vi "Set Exp to test.vi"(0 "Test Information":T1={"Exp Name"="Cold Switching", "Lot"="0233A", "Wafer"="15", "Die Type"="L22", "Die X "="6", "Die Y"="8", "Exp"="1", "Die X_Y"="8"}, 5 "Experiments":T3={"Exp 1"={"P2_Sweep_Stop_V"=36.0, "P2_Sweep_Step_V"=1.0, "Experiment Name"="", "Resistance Threshold"=1.0, "P1_Fixed_Voltage"=36.0, "P2_Sweep_Start_V"=36.0}, "Exp 3"={"P2_Sweep_Stop_V"=36.0, "P2_Sweep_Step_V"=1.0, "Experiment Name"="", "Resistance Threshold"=1.0, "P1_Fixed_Voltage"=36.0, "P2_Sweep_Start_V"=36.0}, "Exp 2"={"P2_Sweep_Stop_V"=36.0, "P2_Sweep_Step_V"=1.0, "Experiment Name"="", "Resistance Threshold"=1.0, "P1_Fixed_Voltage"=36.0, "P2_Sweep_Start_V"=36.0}, "Exp 4"={"P2_Sweep_Stop_V"=36.0, "P2_Sweep_Step_V"=1.0, "Experiment Name"="", "Resistance Threshold"=1.0, "P1_Fixed_Voltage"=36.0, "P2_Sweep_Start_V"=36.0}}, 11 "Error In":errorcluster) -> (4 "Selected Exp Settings":T2={"P2_Sweep_Stop_V"=36.0, "P2_Sweep_Step_V"=1.0, "Experiment Name"="", "Resistance Threshold"=1.0, "P1_Fixed_Voltage"=36.0, "P2_Sweep_Start_V"=36.0}, 6 "Test Information Out":T1={"Exp Name"="Cold Switching", "Lot"="0233A", "Wafer"="15", "Die Type"="L22", "Die X "="6", "Die Y"="8", "Exp"="1", "Die X_Y"="8"}, 15 "Error Out":errorcluster)   [LabVIEW 2013]
uses:
  Controls/Multiple Exp Setup.ctl
  Controls/Individual User Inputs.ctl
  Controls/Test Information.ctl
panel:
  # "Test Settings"
  # "Make the Stop and Step Negative \nfor negative sweep"
  # "Calculation Settings"
  # "Test Settings"
  # "Make the Stop and Step Negative \nfor negative sweep"
  # "Calculation Settings"
  # "Test Settings"
  # "Make the Stop and Step Negative \nfor negative sweep"
  # "Calculation Settings"
  # "Test Settings"
  # "Make the Stop and Step Negative \nfor negative sweep"
  # "Calculation Settings"
  # "Test Settings"
  # "Make the Stop and Step Negative \nfor negative sweep"
  # "Calculation Settings"
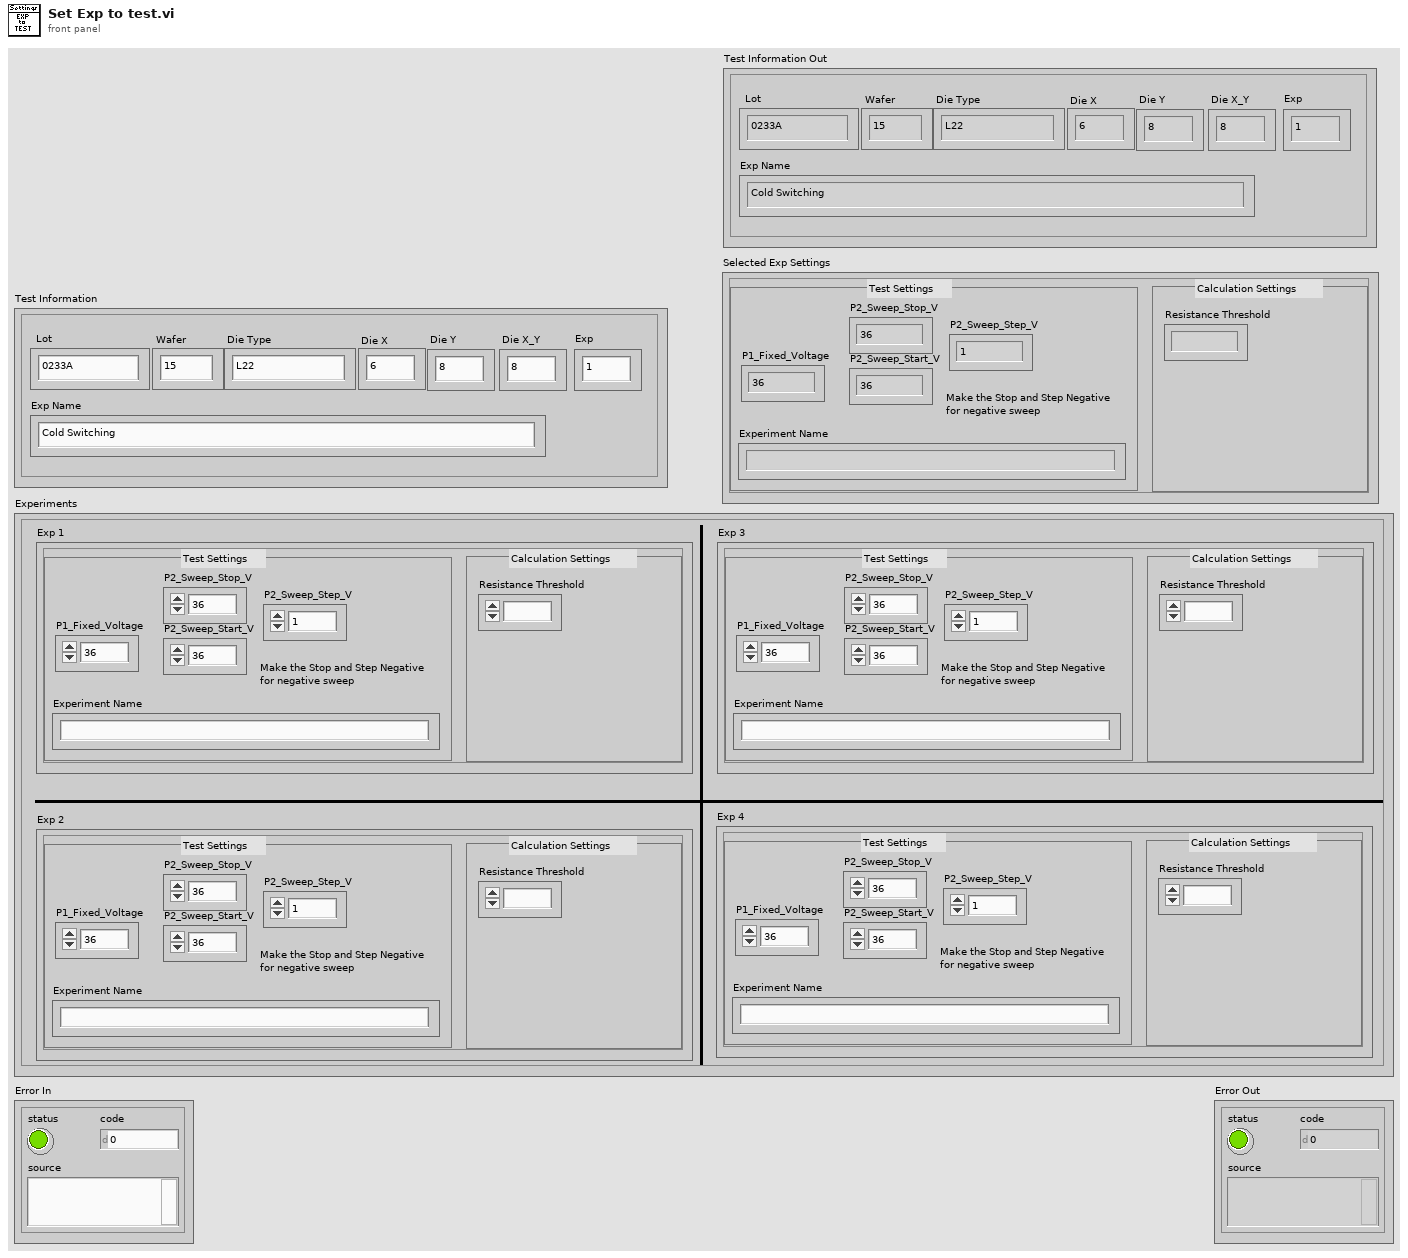
[diagram p1: front panel]
types:
  T1 = typedef "Test Information.ctl" = cluster{"Exp Name":string, "Lot":string, "Wafer":string, "Die Type":string, "Die X ":string, "Die Y":string, "Exp":string, "Die X_Y":string}
  T2 = typedef "Individual User Inputs.ctl" = cluster{"P2_Sweep_Stop_V":dbl, "P2_Sweep_Step_V":dbl, "Experiment Name":string, "Resistance Threshold":dbl, "P1_Fixed_Voltage":dbl, "P2_Sweep_Start_V":dbl}
  T3 = typedef "Multiple Exp Setup.ctl" = cluster{"Exp 1":T2, "Exp 3":T2, "Exp 2":T2, "Exp 4":T2}
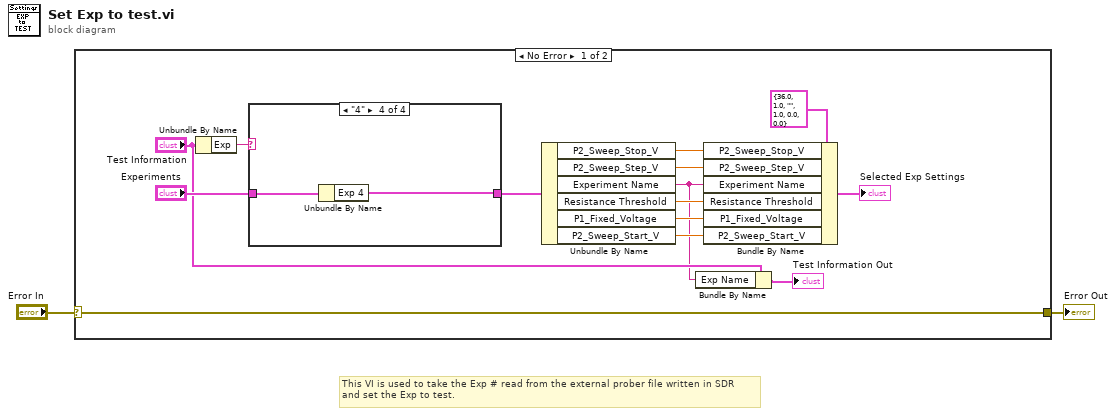
[diagram p0: block diagram]
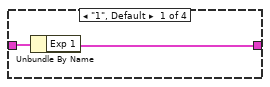
[diagram p2: hidden frame]
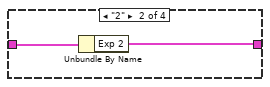
[diagram p3: hidden frame]
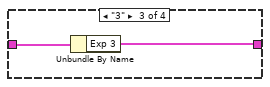
[diagram p4: hidden frame]
diagram:
  # "This VI is used to take the Exp # read from the external prober file written in SDR\nand set the Exp to test."
  n1 = case shown="No Error" "Error In" {
    selector: "Error In" -> [w12 w25]
    tunnel: [w12 w25] -> w1
    frame No Error {
      n2 = Unbundle By Name("Test Information") -> ("Exp"=w16:string)
      n3 = case shown="\"4\"" w16 {
        tunnel: "Experiments" -> [w18 w20 w22 w24]
        tunnel: [w17 w19 w21 w23] -> w4
        frame "1", Default {
          n4 = Unbundle By Name(w18) -> ("Exp 1"=w17:T2)
        }
        frame "2" {
          n5 = Unbundle By Name(w20) -> ("Exp 2"=w19:T2)
        }
        frame "3" {
          n6 = Unbundle By Name(w22) -> ("Exp 3"=w21:T2)
        }
        frame "4" {
          n7 = Unbundle By Name(w24) -> ("Exp 4"=w23:T2)
        }
      }
      n8 = Unbundle By Name(w4) -> ("P2_Sweep_Stop_V"=w9:dbl, "P2_Sweep_Step_V"=w8:dbl, "Experiment Name"=w3:string, "Resistance Threshold"=w7:dbl, "P1_Fixed_Voltage"=w6:dbl, "P2_Sweep_Start_V"=w5:dbl)
      n9 = Bundle By Name(cluster="Test Information", "Exp Name"=w3) -> (→"Test Information Out":T1)
      n10 = Bundle By Name(cluster=T2 {"P2_Sweep_Stop_V"=36.0, "P2_Sweep_Step_V"=1.0, "Experiment Name"="", "Resistance Threshold"=1.0, "P1_Fixed_Voltage"=0.0, "P2_Sweep_Start_V"=0.0} ("Exp"), "P2_Sweep_Stop_V"=w9, "P2_Sweep_Step_V"=w8, "Experiment Name"=w3, "Resistance Threshold"=w7, "P1_Fixed_Voltage"=w6, "P2_Sweep_Start_V"=w5) -> (→"Selected Exp Settings":T2)
    }
    frame Error {
    }
  }
  "Error Out" <- w1
